vi "task5_BINARY2DEC_CONVERTER_SUB_VI.vi"() -> ()   [LabVIEW 2017]
panel:
  out "Tank":dbl(slide) scale=0.0..300.0
  out "Meter":dbl(knob) scale=0.0..300.0
  out "Gauge":dbl(knob) scale=0.0..300.0
  out "display":dbl
  in  "2^0":bool
  in  "2^1":bool
  in  "2^2":bool
  in  "2^3":bool
  in  "2^4":bool
  in  "2^5":bool
  in  "2^6":bool
  in  "2^7":bool
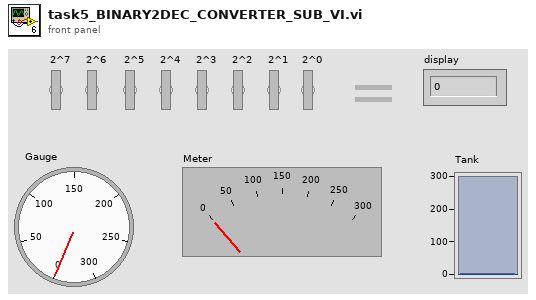
[diagram p1: front panel]
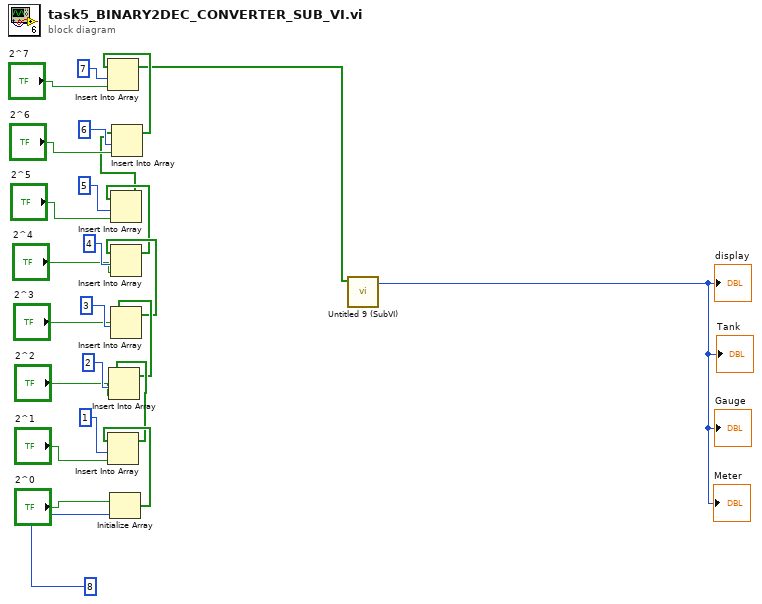
[diagram p0: block diagram]
diagram:
  n1 = Initialize Array("2^0", 8) -> (w8:bool[])
  n2 = Insert Into Array(array=w8, index=1, new element="2^1") -> (w7:bool[])
  n3 = Insert Into Array(array=w7, index=2, new element="2^2") -> (w6:bool[])
  n4 = Insert Into Array(array=w6, index=3, new element="2^3") -> (w5:bool[])
  n5 = Insert Into Array(array=w5, index=4, new element="2^4") -> (w4:bool[])
  n6 = Insert Into Array(array=w4, index=5, new element="2^5") -> (w3:bool[])
  n7 = Insert Into Array(array=w3, index=6, new element="2^6") -> (w2:bool[])
  n8 = Insert Into Array(array=w2, index=7, new element="2^7") -> (w1:bool[])
  n9 = call "Untitled 9 (SubVI).vi"("Array"=w1) -> ("Numeric"=→"display" →"Gauge" →"Meter" →"Tank":i16)  [unwired: 10 in]
